vi "选图.vi"() -> (0 "选鞋数据":string)   [LabVIEW 2018]
uses:
  <vilib>/Utility/file.llb/Read Delimited Spreadsheet (string).vi
panel:
  out "字符串 4":string
  in  "选定鞋":bool
  out "字符串 3":string
  out "表格":string[][](table)
  in  "更新天气情况":bool
  out "字符串 2":string
  out "字符串":string
  in  "前一张":bool
  in  "后一张":bool
  in  "打开":bool
  out "select your shoes":picture
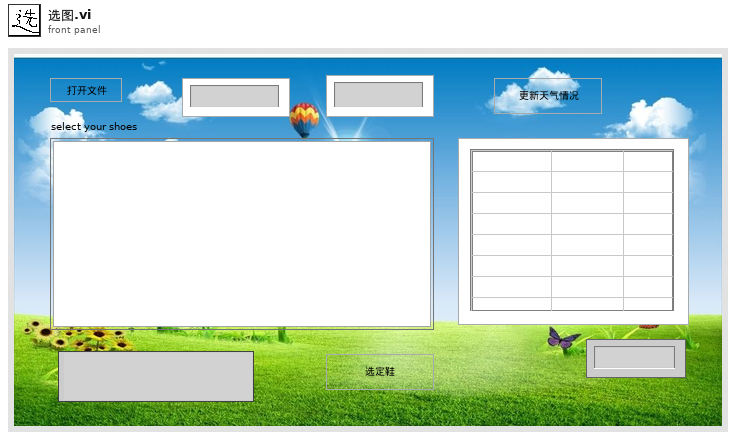
[diagram p1: front panel]
types:
  T1 = typedef "imagedata.ctl" = cluster{"image type":i32, "image depth":i32, "image":u8[], "mask":u8[], "colors":u32[], "Rectangle":cluster{"left":i16, "top":i16, "right":i16, "bottom":i16}}
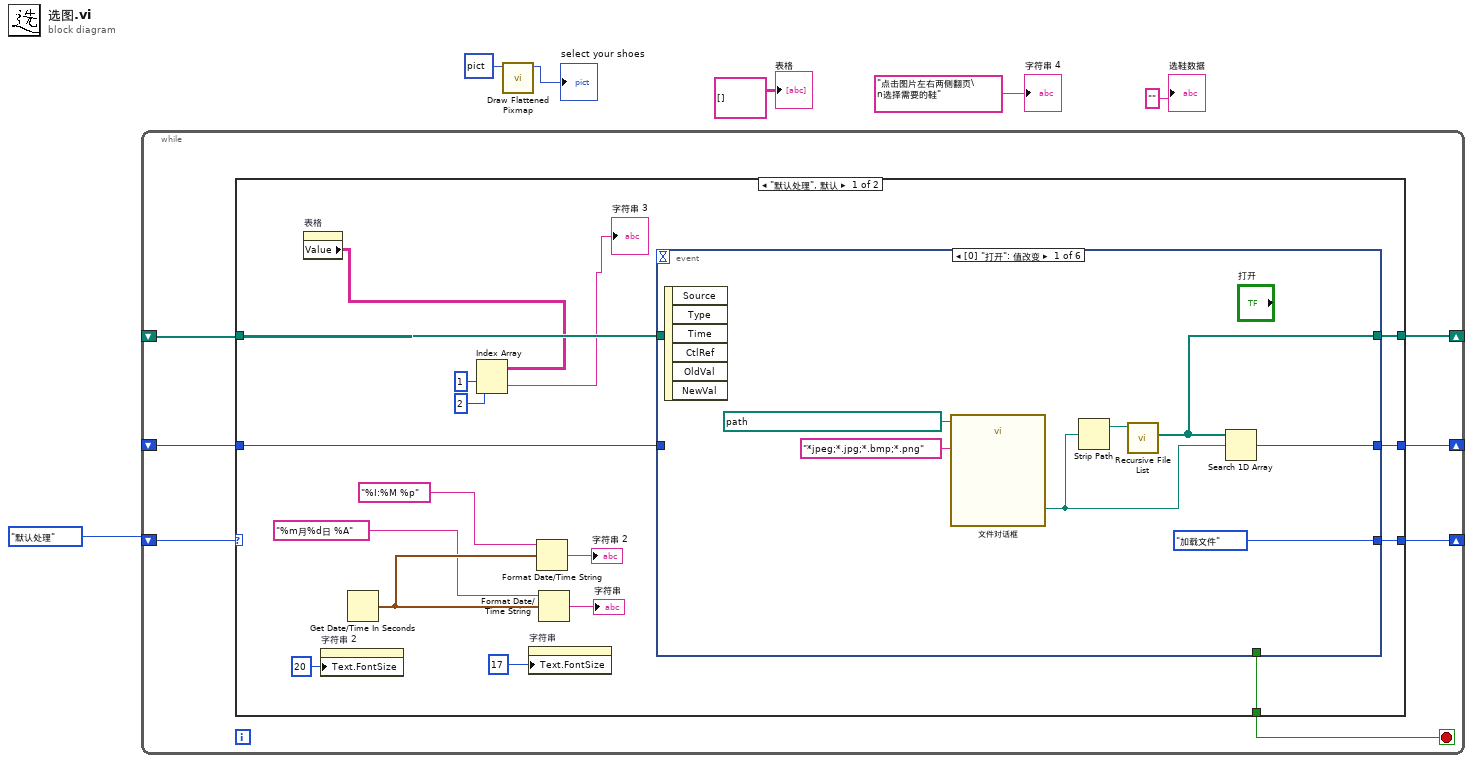
[diagram p0: block diagram]
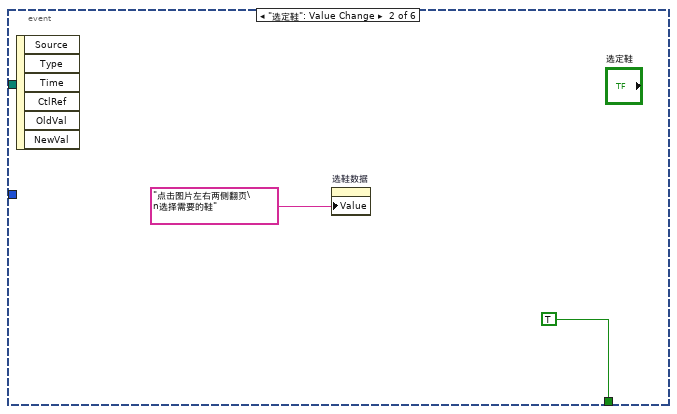
[diagram p2: hidden frame]
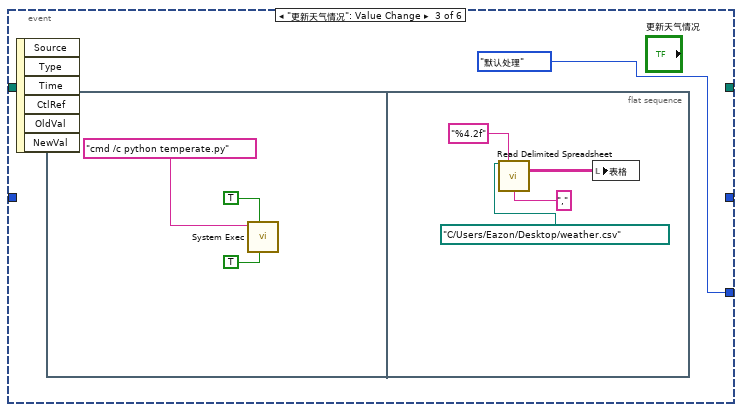
[diagram p3: hidden frame]
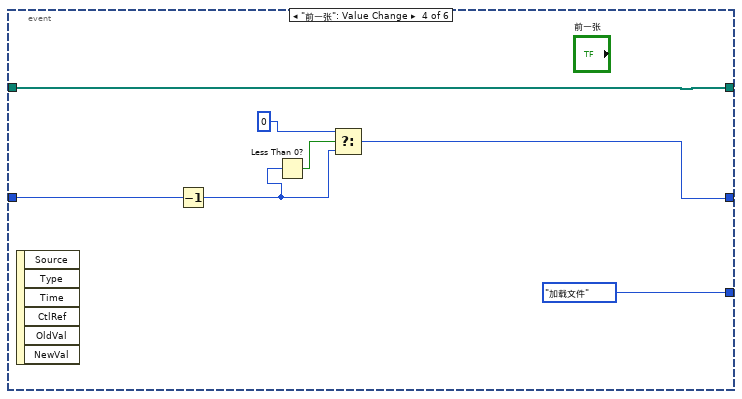
[diagram p4: hidden frame]
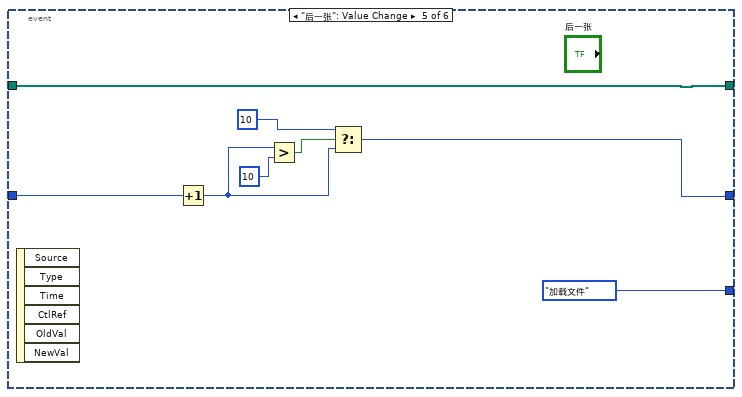
[diagram p5: hidden frame]
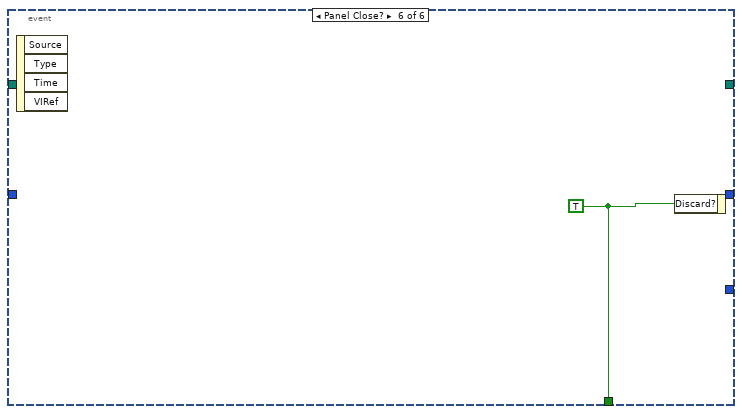
[diagram p6: hidden frame]
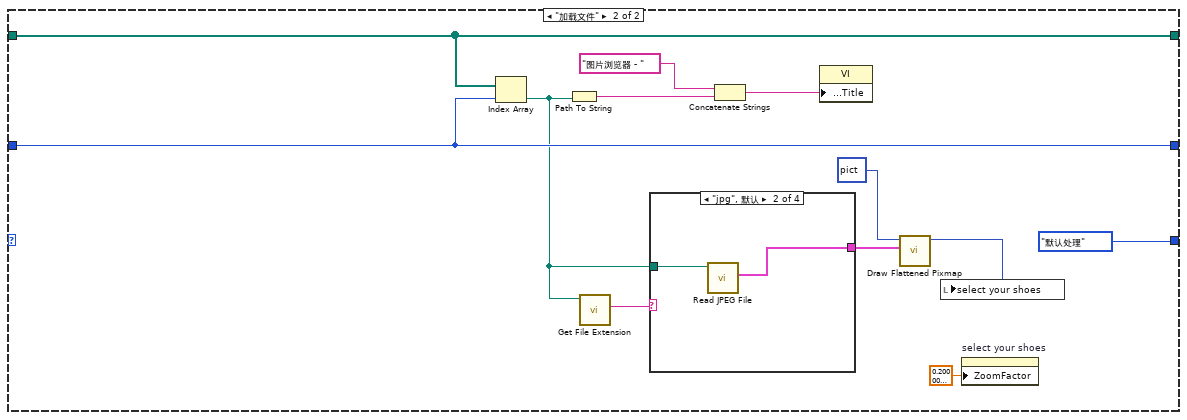
[diagram p7: hidden frame]
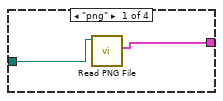
[diagram p8: hidden frame]
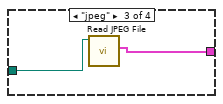
[diagram p9: hidden frame]
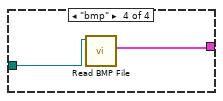
[diagram p10: hidden frame]
diagram:
  n1 = while {
    shift-right: [w13] -> _
    shift-left: _ -> [w11]
    shift-right: [w12] -> _
    shift-left: _ -> [w10]
    shift-right: [w9] -> _
    shift-left: enum16{"默认处理", "加载文件"}."默认处理" -> [w8]
    stop <- w7 stop-if-true
    n2 = case shown="\"默认处理\", 默认" w8 {
      tunnel: [w30 w71] -> w13
      tunnel: [w29 w70] -> w12
      tunnel: w11 -> [w28 w71]
      tunnel: w10 -> [w27 w70]
      tunnel: [w26 enum16{"默认处理", "加载文件"}."默认处理"] -> w9
      tunnel: [w25 _] -> w7
      frame "默认处理", Default {
        n3 = property on="表格" class="Tbl (严格)"() -> ("Value"=w17:string[][])  [unwired: 2 in, 2 out]
        n4 = property on="字符串 2" class="Str"("Text.FontSize"=u32 20 ("文本.字体:字号")) -> ()  [unwired: 2 in, 2 out]
        n5 = Get Date/Time In Seconds() -> (seconds since 1Jan1904=w22:timestamp)
        n6 = Index Array(array=w17, index (row)=1 ("索引 (行)"), index (col)=2 ("禁用的索引 (列)")) -> (element=→"字符串 3":string)
        n7 = property on="字符串" class="Str"("Text.FontSize"=u32 17 ("文本.字体:字号")) -> ()  [unwired: 2 in, 2 out]
        n8 = Format Date/Time String(time format string (%c)="%I:%M %p" ("时间格式字符串(%c)"), seconds (now)=w22) -> (date/time string=→"字符串 2":string)  [unwired: 1 in]
        n9 = Format Date/Time String(time format string (%c)="%m月%d日 %A" ("时间格式字符串(%c)"), seconds (now)=w22) -> (date/time string=→"字符串":string)  [unwired: 1 in]
        n10 = event shown="[0] \"打开\": 值改变" {
          selector: _ -> [_ _ _ _ _ _]
          dyn-events: _ -> [_ _ _ _ _ _]
          timeout: _ -> [_ _ _ _ _ _]
          tunnel: [w34 _ _ w54 w62 _] -> w30
          tunnel: [w33 _ _ w49 w59 _] -> w29
          tunnel: w28 -> [_ _ _ w54 w62 _]
          tunnel: w27 -> [_ _ _ w53 w61 _]
          tunnel: [enum16{"默认处理", "加载文件"}."加载文件" _ enum16{"默认处理", "加载文件"}."默认处理" enum16{"默认处理", "加载文件"}."加载文件" enum16{"默认处理", "加载文件"}."加载文件" _] -> w26
          tunnel: [_ TRUE _ _ _ w63] -> w25
          event "打开": Value Change {
            n11 = event-data() -> ()  [unwired: 1 in, 6 out]
            n12 = call "文件对话框"("start path"=path "E:/操作/labview上位机/智能鞋柜/pics", "pattern (all files)"="*jpeg;*.jpg;*.bmp;*.png") -> ("selected path"=w35:path)  [unwired: 10 in, 3 out]
            n13 = Strip Path(path=w35) -> (stripped path=w36:path)  [unwired: 1 out]
            n14 = call <vilib>:"Recursive File List.vi"("Folder Path"=w36) -> ("All Files in Dir"=w34:path[])  [unwired: 6 in, 4 out]
            n15 = Search 1D Array(1D array=w34, element=w35) -> (index of element=w33:i32)  [unwired: 1 in]
          }
          event "选定鞋": Value Change {
            n16 = event-data() -> ()  [unwired: 1 in, 6 out]
            n17 = property on="选鞋数据" class="Str"("Value"="点击图片左右两侧翻页\n选择需要的鞋" ("选鞋数据")) -> ()  [unwired: 2 in, 2 out]
          }
          event "更新天气情况": Value Change {
            n18 = event-data() -> ()  [unwired: 1 in, 6 out]
            n19 = flat-sequence {
              frame #0 {
                n20 = call <vilib>:"System Exec.vi"("run minimized? (F)"=TRUE, "wait until completion? (T)"=TRUE, "command line"="cmd /c python temperate.py") -> ()  [unwired: 5 in, 4 out]
              }
              frame #1 {
                n21 = call-poly <vilib>:"Read Delimited Spreadsheet.vi"("file path (dialog if empty)"=path "C:/Users/Eazon/Desktop/weather.csv", "format (%s)"="%4.2f" ("format (%.3f)"), "delimiter (\\t)"="," ("delimiter (\\t)")) -> ("all rows"=w47:string[][])  [unwired: 7 in, 5 out]
                n22 = local write "表格"(w47) -> ()
              }
            }
          }
          event "前一张": Value Change {
            n23 = event-data() -> ()  [unwired: 1 in, 6 out]
            n24 = Decrement(x=w53) -> (x-1=w51:i32)
            n25 = Less Than 0?(x=w51) -> (x < 0?=w52:bool)
            n26 = Select(t=0, s=w52, f=w51) -> (s? t:f=w49:i32)
          }
          event "后一张": Value Change {
            n27 = event-data() -> ()  [unwired: 1 in, 6 out]
            n28 = Increment(x=w61) -> (x+1=w56:i32)
            n29 = Greater?(x=w56, y=10) -> (0:w55:bool)
            n30 = Select(t=10, s=w55, f=w56) -> (s? t:f=w59:i32)
          }
          event Panel Close? {
            w63 = TRUE
            n31 = event-data() -> ()  [unwired: 1 in, 4 out]
            n32 = event-data("Discard?"=w63) -> ()  [unwired: 1 in, 1 out]
          }
        }
      }
      frame "加载文件" {
        n33 = Index Array(array=w71, index=w70) -> (element=w69:path)
        n34 = Path To String(path=w69) -> (string=w73:string)
        n35 = call <vilib>:"Get File Extension.vi"("file"=w69) -> ("lowercase file extension"=w67:string)  [unwired: 6 in, 4 out]
        n36 = case shown="\"jpg\", 默认" w67 {
          tunnel: w69 -> [w76 w79 w80 w82]
          tunnel: [w77 w78 w81 w83] -> w68
          frame "png" {
            n37 = call <vilib>:"Read PNG File.vi"("path to PNG file"=w76) -> ("image data"=w77:T1)  [unwired: 8 in, 2 out]
          }
          frame "jpg", Default {
            n38 = call <vilib>:"Read JPEG File.vi"("path to JPEG file"=w79) -> ("image data"=w78:T1)  [unwired: 8 in, 2 out]
          }
          frame "jpeg" {
            n39 = call <vilib>:"Read JPEG File.vi"("path to JPEG file"=w80) -> ("image data"=w81:T1)  [unwired: 8 in, 2 out]
          }
          frame "bmp" {
            n40 = call <vilib>:"Read BMP File.vi"("path to BMP file"=w82) -> ("image data"=w83:T1)  [unwired: 8 in, 2 out]
          }
        }
        n41 = Concatenate Strings("图片浏览器 - " ("字符串"), w73) -> (w65:string)
        n42 = property class="VI"("Front Panel.Title"=w65) -> ()  [unwired: 2 in, 2 out]
        n43 = call <vilib>:"Draw Flattened Pixmap.vi"("image data"=w68, "picture"=picture data[5B]) -> ("new picture"=w74:picture)  [unwired: 7 in]
        n44 = local write "select your shoes"(w74) -> ()
        n45 = property on="select your shoes" class="Pict"("ZoomFactor"=sgl 0.2 ("缩放因子")) -> ()  [unwired: 2 in, 2 out]
      }
    }
  }
  n46 = call <vilib>:"Draw Flattened Pixmap.vi"("picture"=picture data[5B]) -> ("new picture"=→"select your shoes":picture)  [unwired: 8 in]
  "表格" <- string[][] [] ("表格控件")
  "字符串 4" <- "点击图片左右两侧翻页\n选择需要的鞋" ("字符串 4")
  "选鞋数据" <- "" ("选鞋数据")
